vi "Destroy User Events.vi"(8 "error in":errorcluster, 11 "Devices to Load in":refnum<class "Devices to Load.lvclass">) -> (0 "error out":errorcluster, 3 "Devices to Load out":refnum<class "Devices to Load.lvclass">)   [LabVIEW 2018, in "Devices to Load Config Actor.lvlib" / "Devices to Load.lvclass"]
uses:
  Devices to Load.lvclass
  Devices to Load.lvclass/Devices to Load.ctl
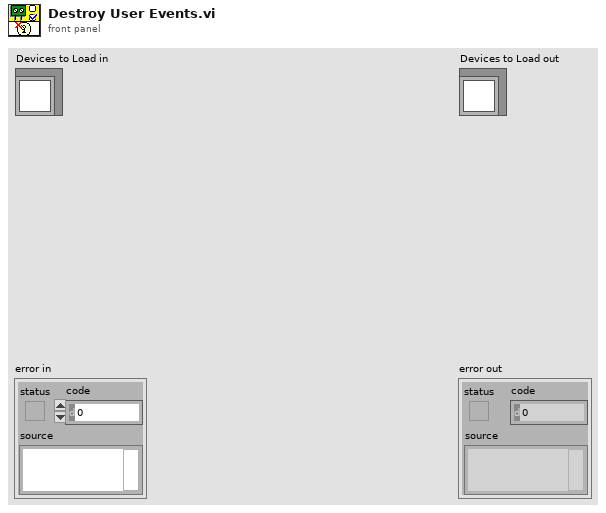
[diagram p1: front panel]
types:
  T1 = typedef "Devices to Load Config Actor.lvlib/Devices to Load.lvclass/Devices to Load User Events.ctl" = cluster{"ItemNames":refnum<user-event>, "stop":refnum<user-event>}
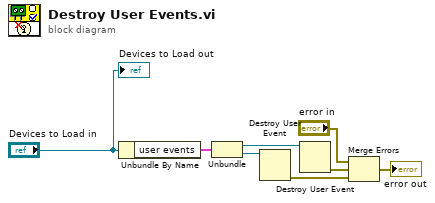
[diagram p0: block diagram]
diagram:
  n1 = Unbundle By Name("Devices to Load in") -> ("user events"=w6:T1)
  n2 = Unbundle(w6) -> ("ItemNames"=w4:refnum<user-event>, "stop"=w5:refnum<user-event>)
  n3 = Destroy User Event(user event=w5) -> (error out=w1:errorcluster)  [unwired: 1 in]
  n4 = Destroy User Event(user event=w4) -> (error out=w2:errorcluster)  [unwired: 1 in]
  n5 = Merge Errors("error in", w2, w1) -> (→"error out":errorcluster)
  "Devices to Load out" <- "Devices to Load in"
